vi "TempReg.vi"() -> ()   [LabVIEW 2014]
panel:
  out "TempDiff":dbl
  in  "stop":bool
  in  "Initial Temperature":dbl
  in  "Heater 2 OFF BUTTON":bool
  out "Garage Temp.":dbl
  out "Garage Temp.":dbl(slide) scale=0.0..110.0
  out "Heater 2 ON":bool
  out "Heater 1 ON":bool
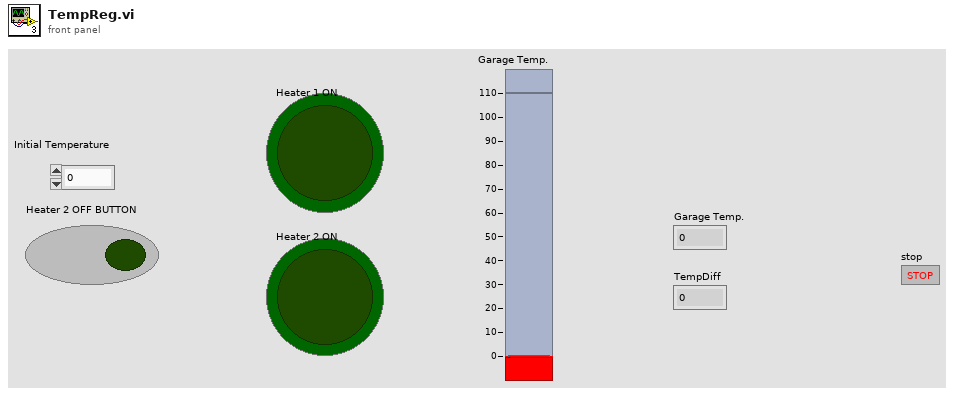
[diagram p1: front panel]
types:
  T1 = enum16{"Both Heaters ON", "Heater 1 ON only", "Both Heaters OFF"}
  T2 = enum16{"Read Temp", "Both Heaters ON", "Heater 1 ON only", "Both Heaters OFF"}
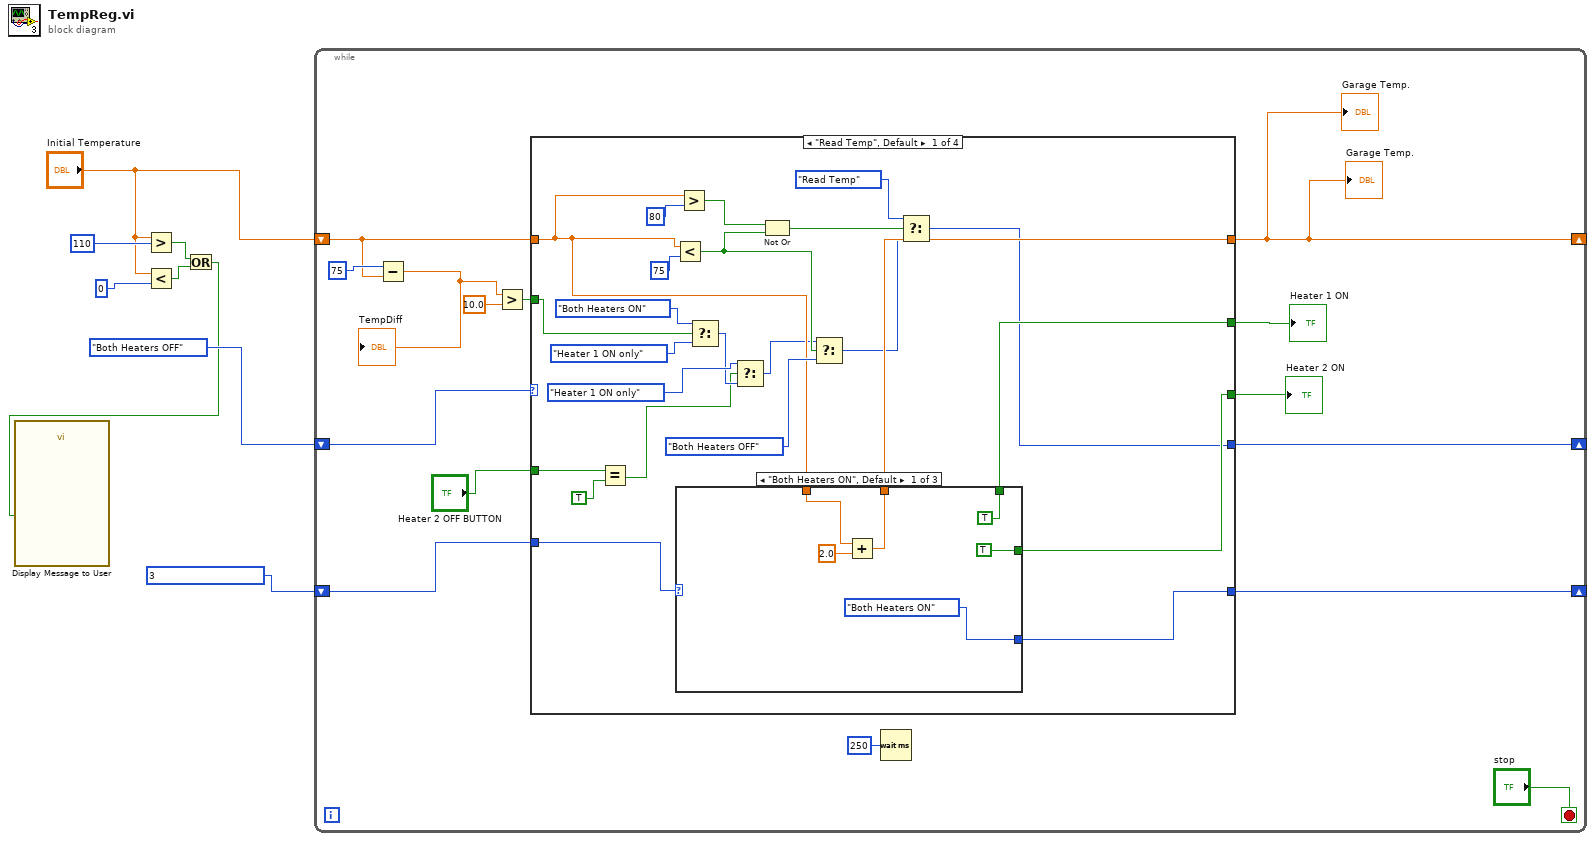
[diagram p0: block diagram]
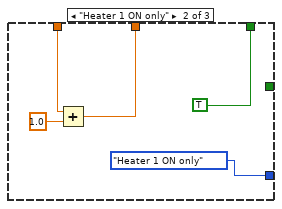
[diagram p2: hidden frame]
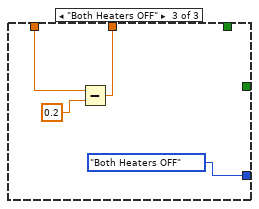
[diagram p3: hidden frame]
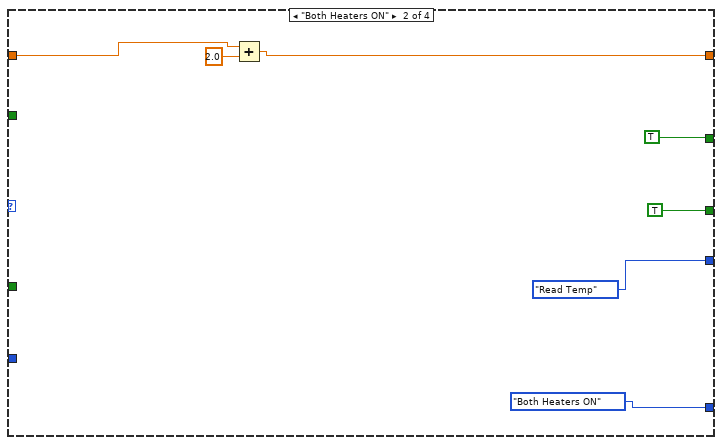
[diagram p4: hidden frame]
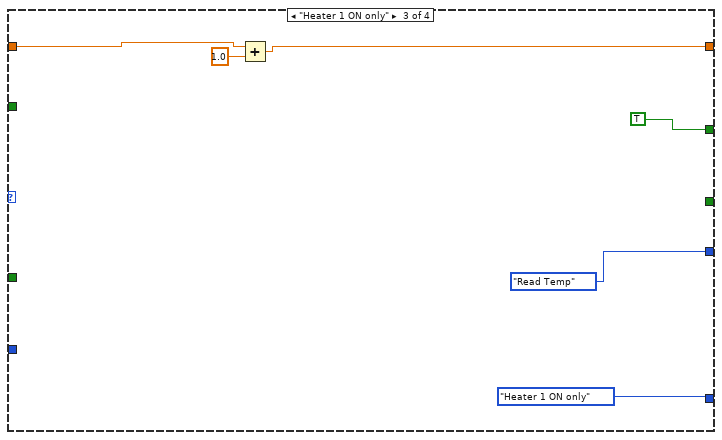
[diagram p5: hidden frame]
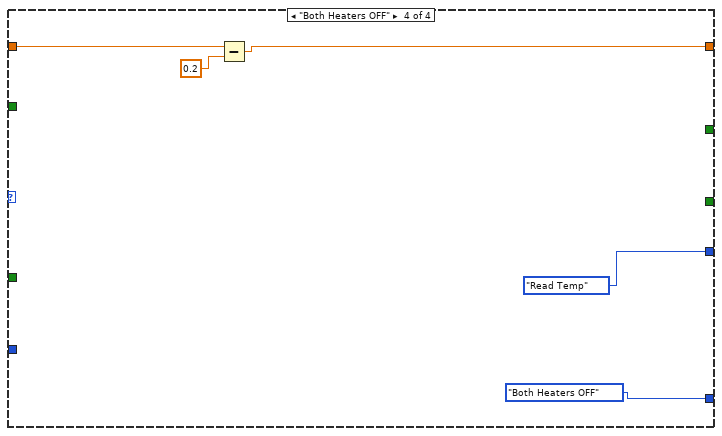
[diagram p6: hidden frame]
diagram:
  n1 = Greater?(x="Initial Temperature", y=110) -> (0:w3:bool)
  n2 = Less?(x="Initial Temperature", y=0) -> (x < y?=w4:bool)
  n3 = Or(x=w3, y=w4) -> (x .or. y?=w1:bool)
  n4 = call "Display Message to User"("Enable"=w1) -> ()  [unwired: 9 in, 2 out]
  n5 = while {
    shift-right: [w20] -> _
    shift-left: T2."Both Heaters OFF" -> [w21]
    shift-right: [w17] -> _
    shift-left: "Initial Temperature" -> [w12]
    shift-right: [w15] -> _
    shift-left: T1 3 -> [w16]
    stop <- "stop" stop-if-true
    n6 = Subtract(x=75, y=w12) -> (x-y=w10:dbl)
    "TempDiff" <- w10
    n7 = Greater?(x=w10, y=10.0) -> (0:w9:bool)
    n8 = case shown="\"Read Temp\", Default" w21 {
      tunnel: w12 -> [w29 w68 w73 w80]
      tunnel: [w44 w67 w72 w78] -> w17
      tunnel: [w24 T2."Read Temp" T2."Read Temp" T2."Read Temp"] -> w20
      tunnel: [w46 TRUE TRUE _] -> w19
      tunnel: [w45 TRUE _ _] -> w18
      tunnel: w16 -> [w47 _ _ _]
      tunnel: [w35 T1."Both Heaters ON" T1."Heater 1 ON only" T1."Both Heaters OFF"] -> w15
      tunnel: "Heater 2 OFF BUTTON" -> [w34 _ _ _]
      tunnel: w9 -> [w31 _ _ _]
      frame "Read Temp", Default {
        n9 = Equal?(x=w34, y=TRUE) -> (x = y?=w26:bool)
        n10 = Less?(x=w29, y=75) -> (x < y?=w37:bool)
        n11 = case shown="\"Both Heaters ON\", Default" w47 {
          tunnel: [TRUE TRUE _] -> w46
          tunnel: [TRUE _ _] -> w45
          tunnel: [w50 w56 w61] -> w44
          tunnel: [T1."Both Heaters ON" T1."Heater 1 ON only" T1."Both Heaters OFF"] -> w35
          tunnel: w29 -> [w48 w54 w59]
          frame "Both Heaters ON", Default {
            n12 = Add(x=w48, y=2.0) -> (x+y=w50:dbl)
          }
          frame "Heater 1 ON only" {
            n13 = Add(x=w54, y=1.0) -> (x+y=w56:dbl)
          }
          frame "Both Heaters OFF" {
            n14 = Subtract(x=w59, y=0.2 ("x-y")) -> (x-y=w61:dbl)
          }
        }
        n15 = Greater?(x=w29, y=80) -> (0:w41:bool)
        n16 = Select(t=T2."Both Heaters ON", s=w31, f=T2."Heater 1 ON only") -> (s? t:f=w27:T2)
        n17 = Select(t=T2."Heater 1 ON only", s=w26, f=w27) -> (s? t:f=w25:T2)
        n18 = Not Or(1:w37, 2:w41) -> (0:w39:bool)
        n19 = Select(t=w25, s=w37, f=T2."Both Heaters OFF") -> (s? t:f=w36:T2)
        n20 = Select(t=T2."Read Temp", s=w39, f=w36) -> (s? t:f=w24:T2)
      }
      frame "Both Heaters ON" {
        n21 = Add(x=w68, y=2.0) -> (x+y=w67:dbl)
      }
      frame "Heater 1 ON only" {
        n22 = Add(x=w73, y=1.0) -> (x+y=w72:dbl)
      }
      frame "Both Heaters OFF" {
        n23 = Subtract(x=w80, y=0.2 ("x-y")) -> (x-y=w78:dbl)
      }
    }
    "Heater 1 ON" <- w19
    "Heater 2 ON" <- w18
    "Garage Temp." <- w17
    "Garage Temp." <- w17
    n24 = Wait (ms)(milliseconds to wait=u32 250) -> ()  [unwired: 1 out]
  }
